vi "Create Ephemeral RSA Key.vi"(5 "Key Length (2048)":i32=2048, 7 "Crypto Provider":T1, 8 "error in (no error)":errorcluster, 9 "Export Policy (allow export)":i32(ring)=1 items=["None"=0, "AllowExport"=1, "AllowPlaintextExport"=2, "AllowArchiving"=4, "AllowPlaintextArchiving"=8], 10 "Key Usage (all usages)":i32(ring)=16777215 items=["None"=0, "Decryption"=1, "Signing"=2, "KeyAgreement"=4, "AllUsages"=16777215]) -> (0 "error out":errorcluster, 3 "CngKey out":refnum<k24>)   [LabVIEW 2021, in "dotNET Crypto Key Management.lvlib"]
doc: "Generates a new, randomly generated private/public key pair."
uses:
  dotNET Crypto Key Management.lvlib
  System.Core
  CNG Provider Type.ctl
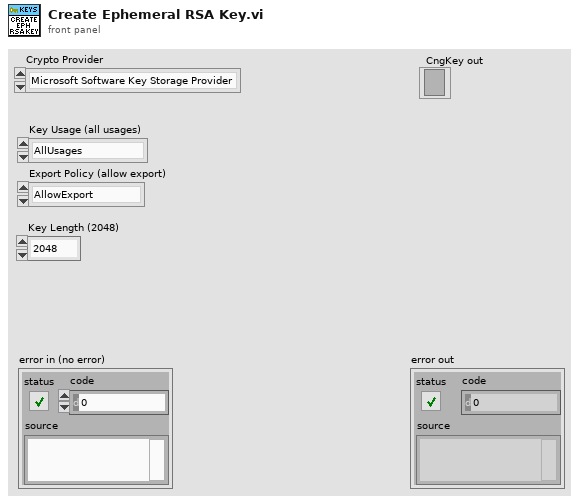
[diagram p1: front panel]
types:
  T1 = typedef "dotNET Crypto Key Management.lvlib/CNG Provider Type.ctl" = enum16{"Microsoft Software Key Storage Provider", "Microsoft Platform Crypto Provider"}
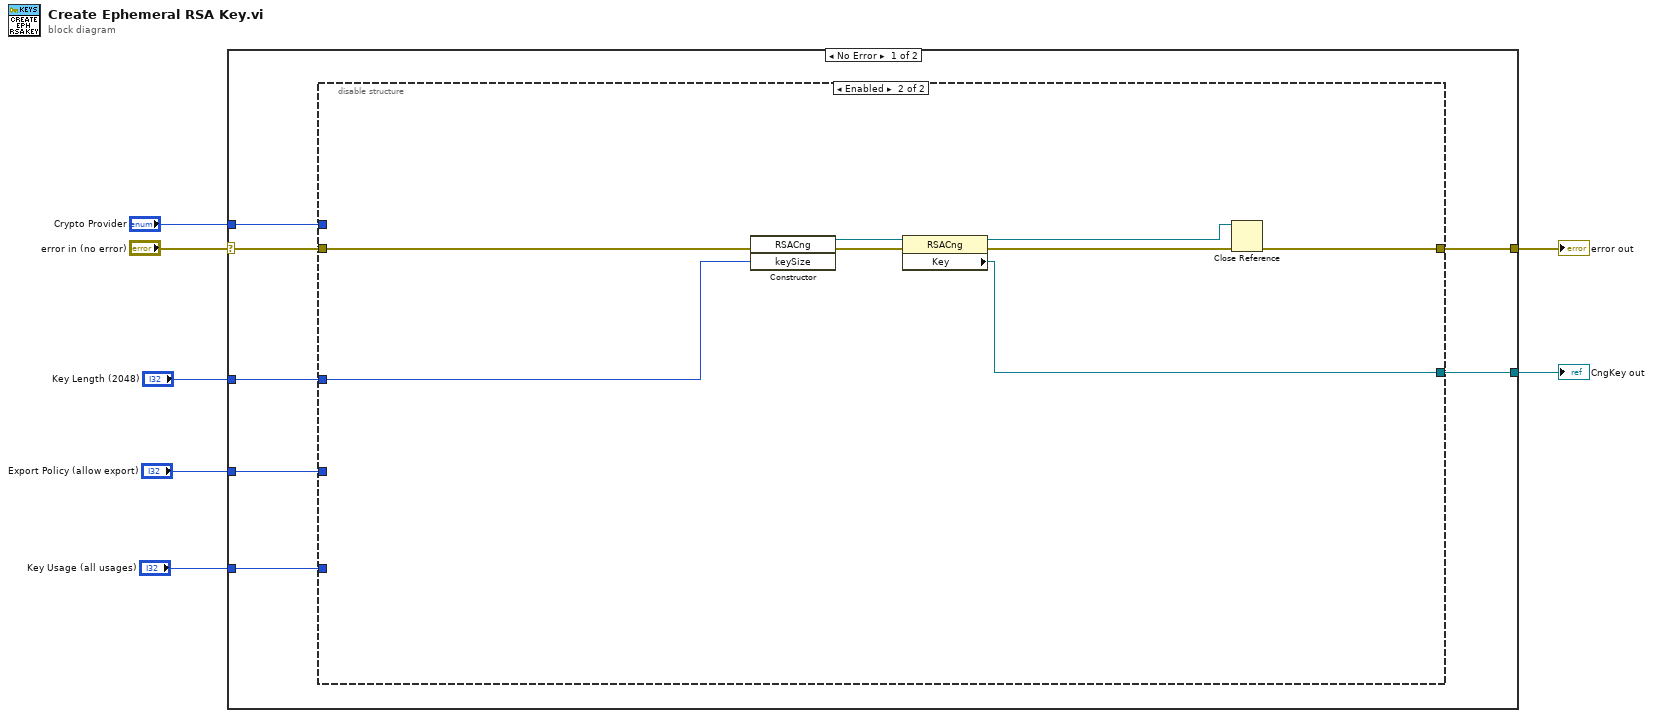
[diagram p0: block diagram]
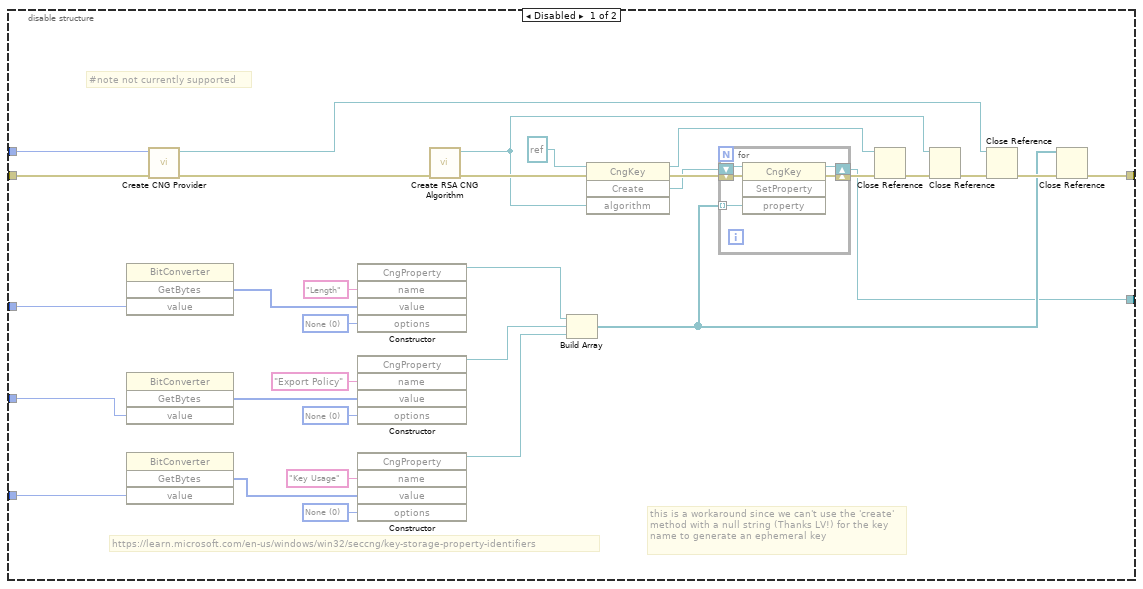
[diagram p2: hidden frame]
diagram:
  n1 = case shown="No Error" "error in (no error)" {
    selector: "error in (no error)" -> [w14 w60]
    tunnel: [w8 _] -> w7
    tunnel: "Export Policy (allow export)" -> [w10 _]
    tunnel: "Crypto Provider" -> [w13 _]
    tunnel: [w11 w60] -> w3
    tunnel: "Key Length (2048)" -> [w12 _]
    tunnel: "Key Usage (all usages)" -> [w9 _]
    frame No Error {
      n2 = disable-structure shown="Enabled" {
        disable-tunnel: w14 -> [w44 w57]
        disable-tunnel: w13 -> [w43 _]
        disable-tunnel: w12 -> [w20 w52]
        disable-tunnel: [w35 w53] -> w11
        disable-tunnel: w10 -> [w18 _]
        disable-tunnel: w9 -> [w16 _]
        disable-tunnel: [w21 w56] -> w8
        frame Disabled {
          w27 = 0 items=["None"=0, "CustomProperty"=1073741824, "Persist"=-2147483648] ("options")
          w30 = 0 items=["None"=0, "CustomProperty"=1073741824, "Persist"=-2147483648] ("options")
          w36 = 0 items=["None"=0, "CustomProperty"=1073741824, "Persist"=-2147483648] ("options")
          # "#note not currently supported"
          # "this is a workaround since we can't use the 'create' method with a null string (Thanks LV!) for the key name to generate an ephemeral key"
          # "https://learn.microsoft.com/en-us/windows/win32/seccng/key-storage-property-identifiers"
          n3 = invoke class="BitConverter" method="GetBytes"("value"=w20) -> ("GetBytes"=w19:u8[])  [unwired: 3 in, 3 out]
          n4 = invoke class="BitConverter" method="GetBytes"("value"=w18) -> ("GetBytes"=w17:u8[])  [unwired: 3 in, 3 out]
          n5 = invoke class="BitConverter" method="GetBytes"("value"=w16) -> ("GetBytes"=w15:u8[])  [unwired: 3 in, 3 out]
          n6 = call "Create CNG Provider.vi"("error in (no error)"=w44, "Crypto Provider"=w43) -> ("error out"=w26:errorcluster, "CngProvider"=w40:refnum<k24>)  [unwired: 8 in]
          n7 = constructor class="CngProperty"("name"="Length", "value"=w19, "options"=w36) -> (reference out=w25:refnum<k24>)  [unwired: 3 in, 5 out]
          n8 = constructor class="CngProperty"("name"="Export Policy", "value"=w17, "options"=w30) -> (reference out=w23:refnum<k24>)  [unwired: 3 in, 5 out]
          n9 = constructor class="CngProperty"("name"="Key Usage", "value"=w15, "options"=w27) -> (reference out=w22:refnum<k24>)  [unwired: 3 in, 5 out]
          n10 = call "Create RSA CNG Algorithm.vi"("error in (no error)"=w26) -> ("error out"=w45:errorcluster, "RSA Cng Algorithm"=w42:refnum<k24>)  [unwired: 9 in]
          n11 = Build Array(w25, w23, w22) -> (w24:refnum<k24>[])
          n12 = invoke class="CngKey" method="Create"(reference=refnum<k24> refnum, error in=w45, "algorithm"=w42) -> (reference out=w31:refnum<k24>, error out=w34:errorcluster, "Create"=w32:refnum<k24>)  [unwired: 1 in, 1 out]
          n13 = for {
            tunnel: w24 -> [w48] mode=indexing
            shift-right: [w50] -> w33
            shift-left: w34 -> [w51]
            shift-right: [w47] -> w21
            shift-left: w32 -> [w49]
            n14 = invoke class="CngKey" method="SetProperty"(reference=w49, error in=w51, "property"=w48) -> (reference out=w47:refnum<k24>, error out=w50:errorcluster)  [unwired: 1 in, 2 out]
          }
          n15 = Close Reference(reference=w31, error in (no error)=w33) -> (error out=w39:errorcluster)
          n16 = Close Reference(reference=w42, error in (no error)=w39) -> (error out=w41:errorcluster)
          n17 = Close Reference(reference=w40, error in (no error)=w41) -> (error out=w38:errorcluster)
          n18 = Close Reference(reference=w24, error in (no error)=w38) -> (error out=w35:errorcluster)
        }
        frame Enabled {
          n19 = constructor class="RSACng"(error in=w57, "keySize"=w52) -> (reference out=w58:refnum<k24>, error out=w59:errorcluster)  [unwired: 2 in, 2 out]
          n20 = property class="RSACng"(reference=w58, error in=w59) -> (reference out=w54:refnum<k24>, error out=w55:errorcluster, "Key"=w56:refnum<k24>)
          n21 = Close Reference(reference=w54, error in (no error)=w55) -> (error out=w53:errorcluster)
        }
      }
    }
    frame Error {
    }
  }
  "error out" <- w3
  "CngKey out" <- w7
